vi "write_DAQ_ex.vi"() -> ()   [LabVIEW 2019]
panel:
  in  "Numeric 2":dbl
  in  "Numeric":dbl
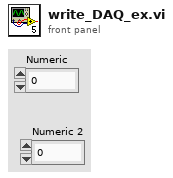
[diagram p1: front panel]
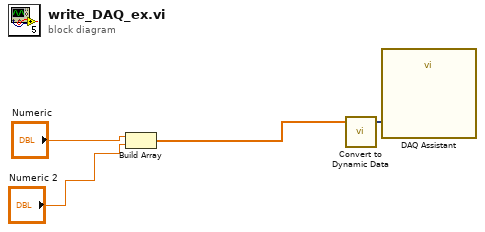
[diagram p0: block diagram]
diagram:
  n1 = Build Array("Numeric", "Numeric 2") -> (w2:dbl[])
  n2 = call "Convert to Dynamic Data"("Array"=w2) -> ("Dynamic Data Type"=w1:dynamicdata)  [unwired: 3 in]
  n3 = call "DAQ Assistant"("data"=w1) -> ()  [unwired: 17 in, 2 out]
